vi "Get Logarithm Range.vi"(9 "Logarithm?":bool, 11 "Range In":cluster{"Max X":sgl, "Min X":sgl}) -> (3 "Range Out":cluster{"Max":sgl, "Min":sgl})   [LabVIEW 2020, in "3D Plot.lvclass"]
uses:
  <vilib>/Math Plots/3D Math Plots/3D Plot/3D Plot/3D Plot.lvclass
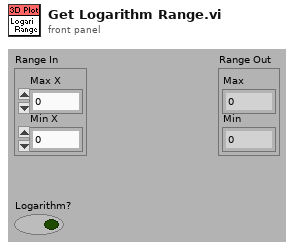
[diagram p1: front panel]
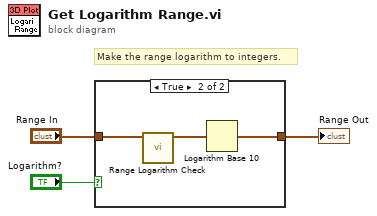
[diagram p0: block diagram]
diagram:
  # "Make the range logarithm to integers."
  n1 = case shown="True" "Logarithm?" {
    tunnel: "Range In" -> [w4 w7]
    tunnel: [w4 w5] -> w2
    frame False {
    }
    frame True {
      n2 = call <vilib>:"Range Logarithm Check.vi"("Logarithm Range In"=w7) -> ("Logarithm Range Out"=w6:cluster{"Max":sgl, "Min":sgl})  [unwired: 10 out]
      n3 = Logarithm Base 10(1:w6) -> (0:w5:cluster{"Max":sgl, "Min":sgl})
    }
  }
  "Range Out" <- w2
